vi "CalcParams.vi"(0 "ClkRate":dbl format="%#_13g", 5 "dT":dbl caption="dT (in sec)" format="%#_13g", 7 "TicksPerRev":u32) -> (4 "dT":u32 caption="dT (in Ticks)", 6 "dTPerSec":dbl, 8 "RevPerPulse":dbl)   [LabVIEW 2015, in "QuadEncInterface.lvlib"]
uses:
  QuadEncInterface.lvlib
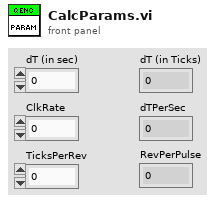
[diagram p1: front panel]
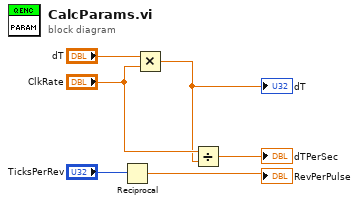
[diagram p0: block diagram]
diagram:
  n1 = Reciprocal(x="TicksPerRev") -> (1/x=→"RevPerPulse":dbl)
  n2 = Multiply(x="dT", y="ClkRate") -> (x*y=w3:dbl)
  "dT" <- w3
  n3 = Divide(x="ClkRate", y=w3) -> (x/y=→"dTPerSec":dbl)
